vi "AI Block Config Pane.vi"(6 "_SubPanelMessages":refnum<notifier>, 9 "_myEmbeddedToFrameEvent":T7, 10 "_myEmbedded.Exit":refnum<user-event>, 11 "-Property Bundle":cluster{"Name":string, "Value":variant}[](array[cluster])) -> (1 "_Connection Informations":T3, 2 "_Scripter Input":T9)   [LabVIEW 2021]
doc: "Reads values from one or more analog input channels. Use this Express VI to read one or multiple samples for each channel at one time."
uses:
  <vilib>/myRIO/Common/Express VI Framework/xctls/myRIO Channel List/myRIO Channel List.xctl
  <vilib>/myRIO/Common/Express VI Framework/typedefs/Config Pane to Framework Ref.ctl
  <vilib>/myRIO/Common/Express VI Framework/typedefs/Data Validate Ref.ctl
  <vilib>/myRIO/Common/Express VI Framework/typedefs/Scripter Input.ctl
  <vilib>/myRIO/Common/Express VI Framework/typedefs/WireThrough Terminal Names.ctl
  <vilib>/myRIO/Common/Express VI Framework/typedefs/Instrument Driver Method Descriptor Array.ctl
  <vilib>/myRIO/Common/Express VI Framework/typedefs/Instrument Driver Method Descriptor.ctl
  <vilib>/myRIO/Common/Express VI Framework/typedefs/Sub Panel Messages.ctl
  <vilib>/myRIO/Common/Express VI Framework/typedefs/Connection Informations.ctl
  <vilib>/myRIO/Common/Instrument Driver Framework/Utilities/typedefs/Channel Types.ctl
  <vilib>/myRIO/Common/Express VI Framework/vis/Express VI Framework Strings Global.vi
panel:
  in  "Range Indexes":i32[](array[numeric])
  in  "Sample Rate Unit":string="kHz"
  out "_learnMoreLatency":string="Gaps exist between sequential n samples acquisitions. Learn more"
  out "_learnMoreFrequency":string="Detailed information about valid sample rates for this Express VI. Learn more"
  in  "_Validate":bool
  in  "Sample Rate:":dbl=1.0 caption="Sample rate:"
  in  "Samples to Read:":u32=1000 caption="Samples:" min=1 max=10000
  in  "Name:":string="Analog input (n samples)" caption="Node name:"
  in  "Selected Channel List":T1[](xcontrol)=[{"Channel Name"=0, "Channel Alias"="", "Remove Channel"=FALSE, "Index"=0}]
  in  "_Default Alias String":string
  in  "_VI Default Name (Edit and make value default)":string="Analog input (n samples)"
  in  "_WireThrough Info (Edit and make value default)":T4={"WireThrough Top In"="AI (N Samples) Ref In", "WireThrough Bottom In"="error in (no error)", "WireThrough Top Out"="AI (N Samples) Ref Out", "WireThrough Bottom Out"="error out"}
  in  "_Template Array (Edit and make value default)":T5=[{"Function Name"="Smart Open", "VI Path"=path "<vilib>/myRIO/Instrument Drivers/Onboard IO/AI Block/vis", "Script"=TRUE, "Inputs"=[{"name"="Channel Names", "value"=variant, "Config Pane Only"=TRUE, "Build Array"=FALSE, "Bundle Cluster"=FALSE, "Show Term"=FALSE, "alias"=[], "Required Input"=FALSE}], "Outputs"=[], "VI Class"=enum."Open", "Controls Refs[]"=[], "Inline"=FALSE}, {"Function Name"="Open", "VI Path"=path "<vilib>/myRIO/Instrument Drivers/Onboard IO/AI Block/vis", "Script"=FALSE, "Inputs"=[{"name"="Channel Names", "value"=variant, "Config Pane Only"=TRUE, "Build Array"=FALSE, "Bundle Cluster"=FALSE, "Show Term"=FALSE, "alias"=[], "Required Input"=FALSE}], "Outputs"=[], "VI Class"=enum."Open", "Controls Refs[]"=[], "Inline"=FALSE}, {"Function Name"="Read", "VI Path"=path "<vilib>/myRIO/Instrument Drivers/Onboard IO/AI Block/vis", "Script"=TRUE, "Inputs"=[{"name"="Number of Samples", "value"=variant, "Config Pane Only"=TRUE, "Build Array"=FALSE, "Bundle Cluster"=FALSE, "Show Term"=FALSE, "alias"=[], "Required Input"=FALSE}, {"name"="Sample Rate [Hz]", "value"=variant, "Config Pane Only"=TRUE, "Build Array"=FALSE, "Bundle Cluster"=FALSE, "Show Term"=FALSE, "alias"=[], "Required Input"=FALSE}], "Outputs"=[{"name"="Values", "value"=variant, "Show Term"=TRUE, "Index Array"=TRUE, "Unbundle Cluster"=FALSE, "alias"=[]}], "VI Class"=enum."Data", "Controls Refs[]"=[], "Inline"=FALSE}, {"Function Name"="Close", "VI Path"=path "<vilib>/myRIO/Instrument Drivers/Onboard IO/AI Block/vis", "Script"=FALSE, "Inputs"=[], "Outputs"=[], "VI Class"=enum."Close", "Controls Refs[]"=[], "Inline"=FALSE}]
  in  "_Test Close":bool
  # "User Visible Area"
  # "NOTE: Tab Order has been set\nfor this Front Panel.\n1. Name: (string control)\n2. Add Channel (button)\n3. Selected Channel List (array)\n\nAll other controls are excluded \nfrom Tabbing order\n\nTo exlude a control from context\nhelp prefix its label text with a '-'"
  # "kHz"
  # "Gap:"
  # "Acquired signal"
  # "Missed signal"
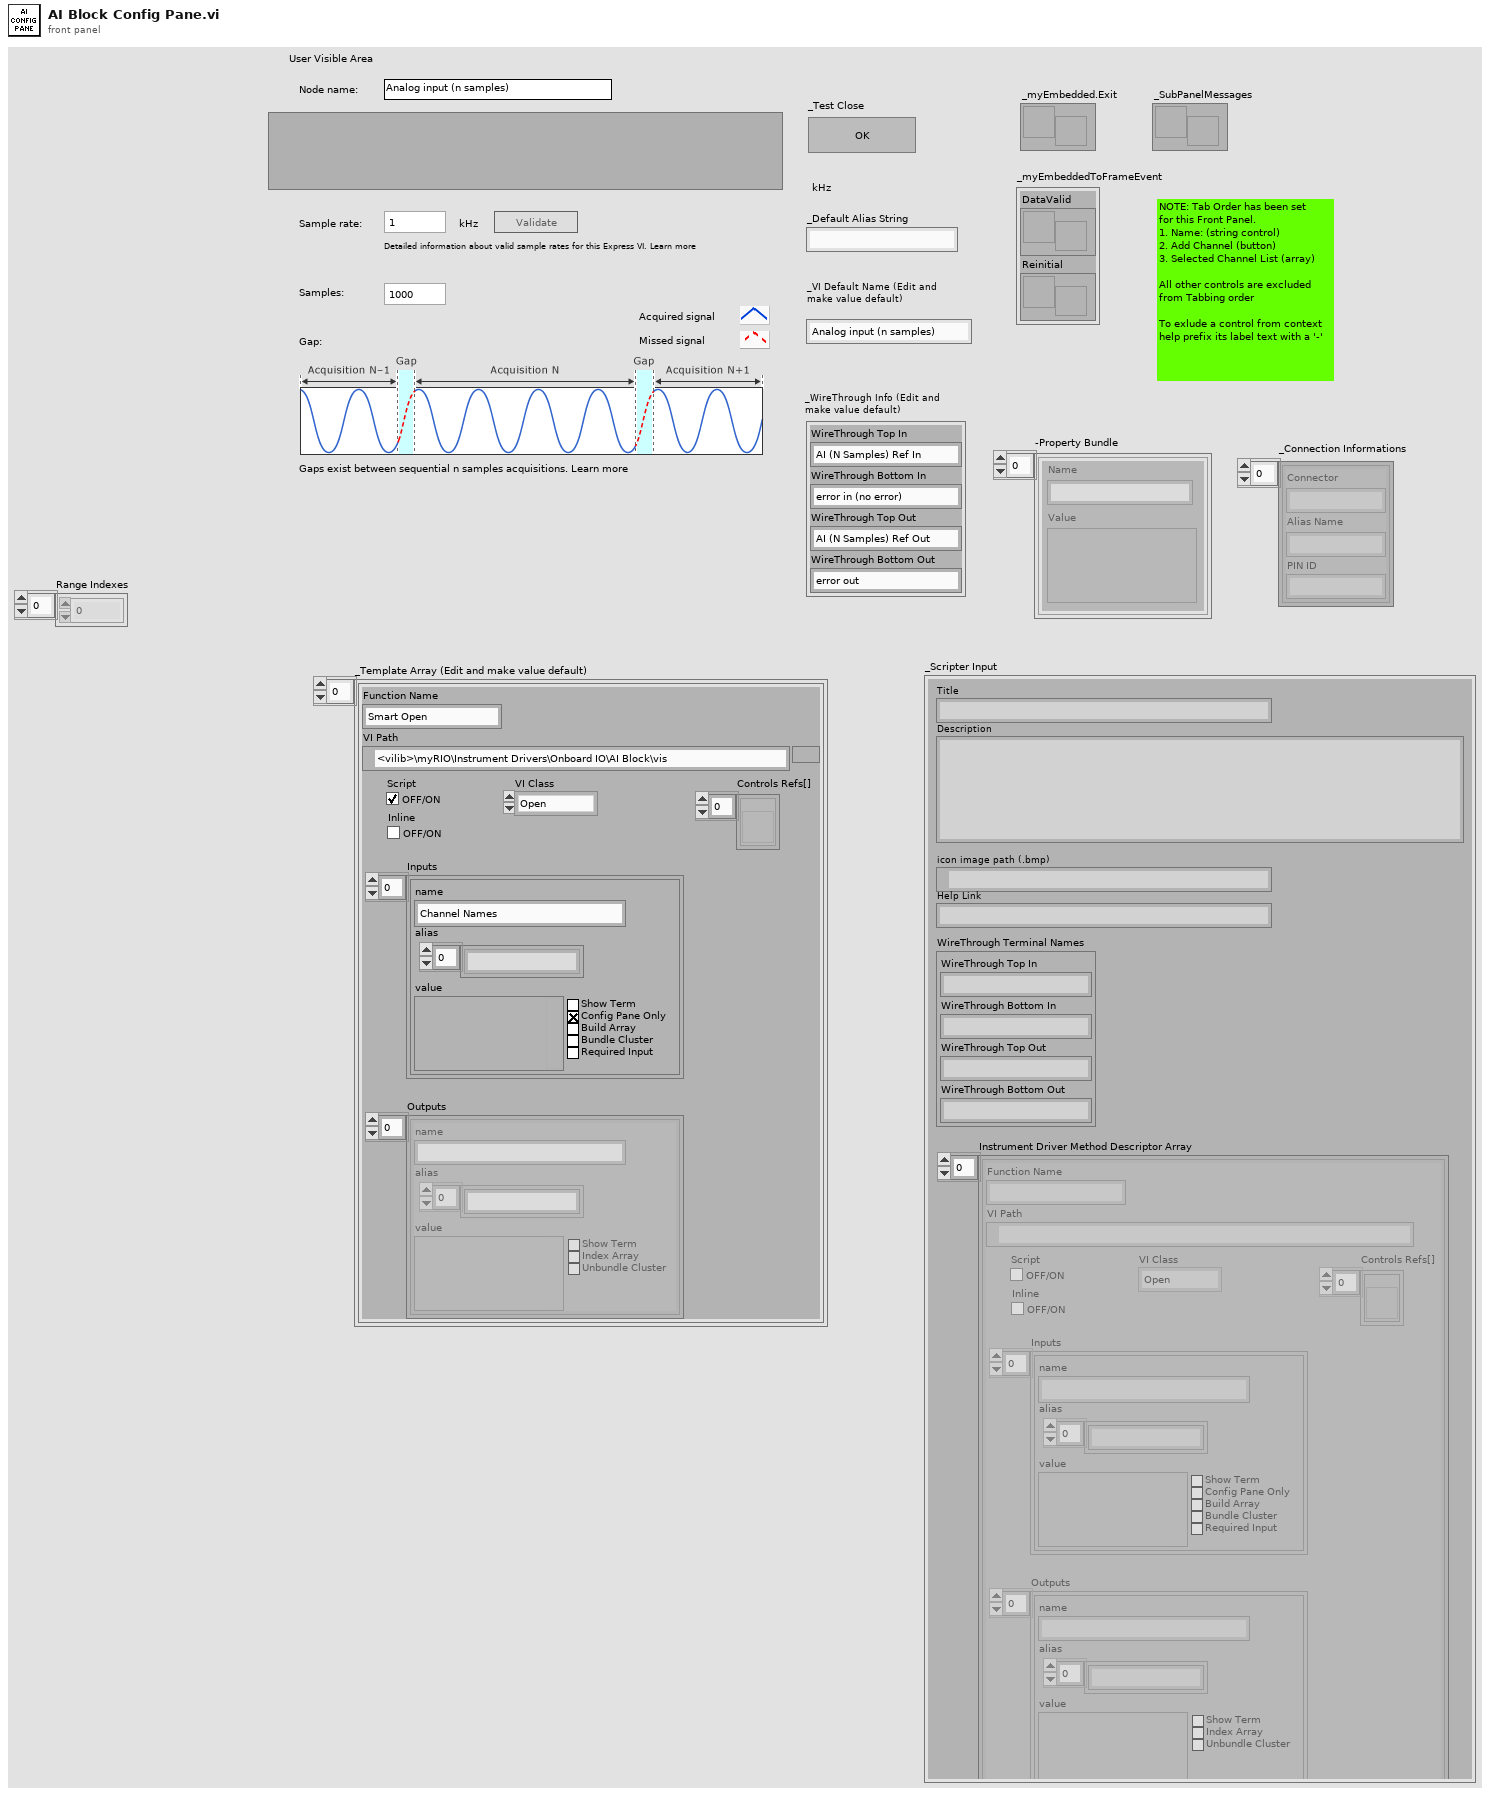
[diagram p1: front panel]
types:
  T1 = typedef "myRIO Channel List.xctl/Channel Data.ctl" = cluster{"Channel Name":u16, "Channel Alias":string, "Remove Channel":T2, "Index":i32}
  T2 = typedef "myRIO Channel List.xctl/Remove Channel.ctl" = bool
  T3 = typedef "Connection Informations.ctl" = cluster{"Connector":string, "Alias Name":string, "PIN ID":string}[]
  T4 = typedef "WireThrough Terminal Names.ctl" = cluster{"WireThrough Top In":string, "WireThrough Bottom In":string, "WireThrough Top Out":string, "WireThrough Bottom Out":string}
  T5 = typedef "Instrument Driver Method Descriptor Array.ctl" = T6[]
  T6 = typedef "Instrument Driver Method Descriptor.ctl" = cluster{"Function Name":string, "VI Path":path, "Script":bool, "Inputs":cluster{"name":string, "value":variant, "Config Pane Only":bool, "Build Array":bool, "Bundle Cluster":bool, "Show Term":bool, "alias":string[], "Required Input":bool}[], "Outputs":cluster{"name":string, "value":variant, "Show Term":bool, "Index Array":bool, "Unbundle Cluster":bool, "alias":string[]}[], "VI Class":enum16{"Open", "Configure", "Data", "Manage", "Close"}, "Controls Refs[]":refnum<vi>[], "Inline":bool}
  T7 = typedef "Config Pane to Framework Ref.ctl" = cluster{"DataValid":T8, "Reinitial":refnum<user-event>}
  T8 = typedef "Data Validate Ref.ctl" = refnum<user-event>
  T9 = typedef "Scripter Input.ctl" = cluster{"Title":string, "Description":string, "icon image path (.bmp)":path, "Help Link":string, "WireThrough Terminal Names":T4, "Instrument Driver Method Descriptor Array":T5}
  T10 = typedef "Channel Types.ctl" = enum32{"Unknown", "AI", "AO", "DIO - DI", "DIO", "DIO - DO", "I2C", "PWM", "Encoder", "SPI", "UART", "Accelerometer", "DIO - LED", "DIO - Button", "AI (N Samples)", "AudioIn (N Samples)", "AO (N Samples)", "AudioOut (N Samples)", "DI (N Samples)", "DO (N Samples)", "AI IRQ", "DI IRQ", "Timer IRQ", "RSL", "Relay", "CAN", "AI (Continuous)", "AO (Continuous)"}
  T11 = typedef "Channel Info.ctl" = cluster{"Channel Name":string, "Alias":string, "Used?":bool, "Not Support?":bool, "Property Bundle":cluster{"Name":string, "Value":variant}[]}
  T12 = typedef "Sub Panel Messages.ctl" = enum16{"Initialized"}
  T13 = enum8{"Enabled", "Disabled", "Disabled and Grayed Out"}
  T14 = cluster{"name":string, "value":variant, "Config Pane Only":bool, "Build Array":bool, "Bundle Cluster":bool, "Show Term":bool, "alias":string[], "Required Input":bool}
  T15 = cluster{"Connector":string, "Alias Name":string, "PIN ID":string}[]
  T16 = cluster{"name":string, "value":variant, "Config Pane Only":bool, "Build Array":bool, "Bundle Cluster":bool, "Show Term":bool, "alias":string[], "Required Input":bool}[]
  T17 = cluster{"name":string, "value":variant, "Show Term":bool, "Index Array":bool, "Unbundle Cluster":bool, "alias":string[]}[]
  T18 = cluster{"name":string, "value":variant, "Show Term":bool, "Index Array":bool, "Unbundle Cluster":bool, "alias":string[]}
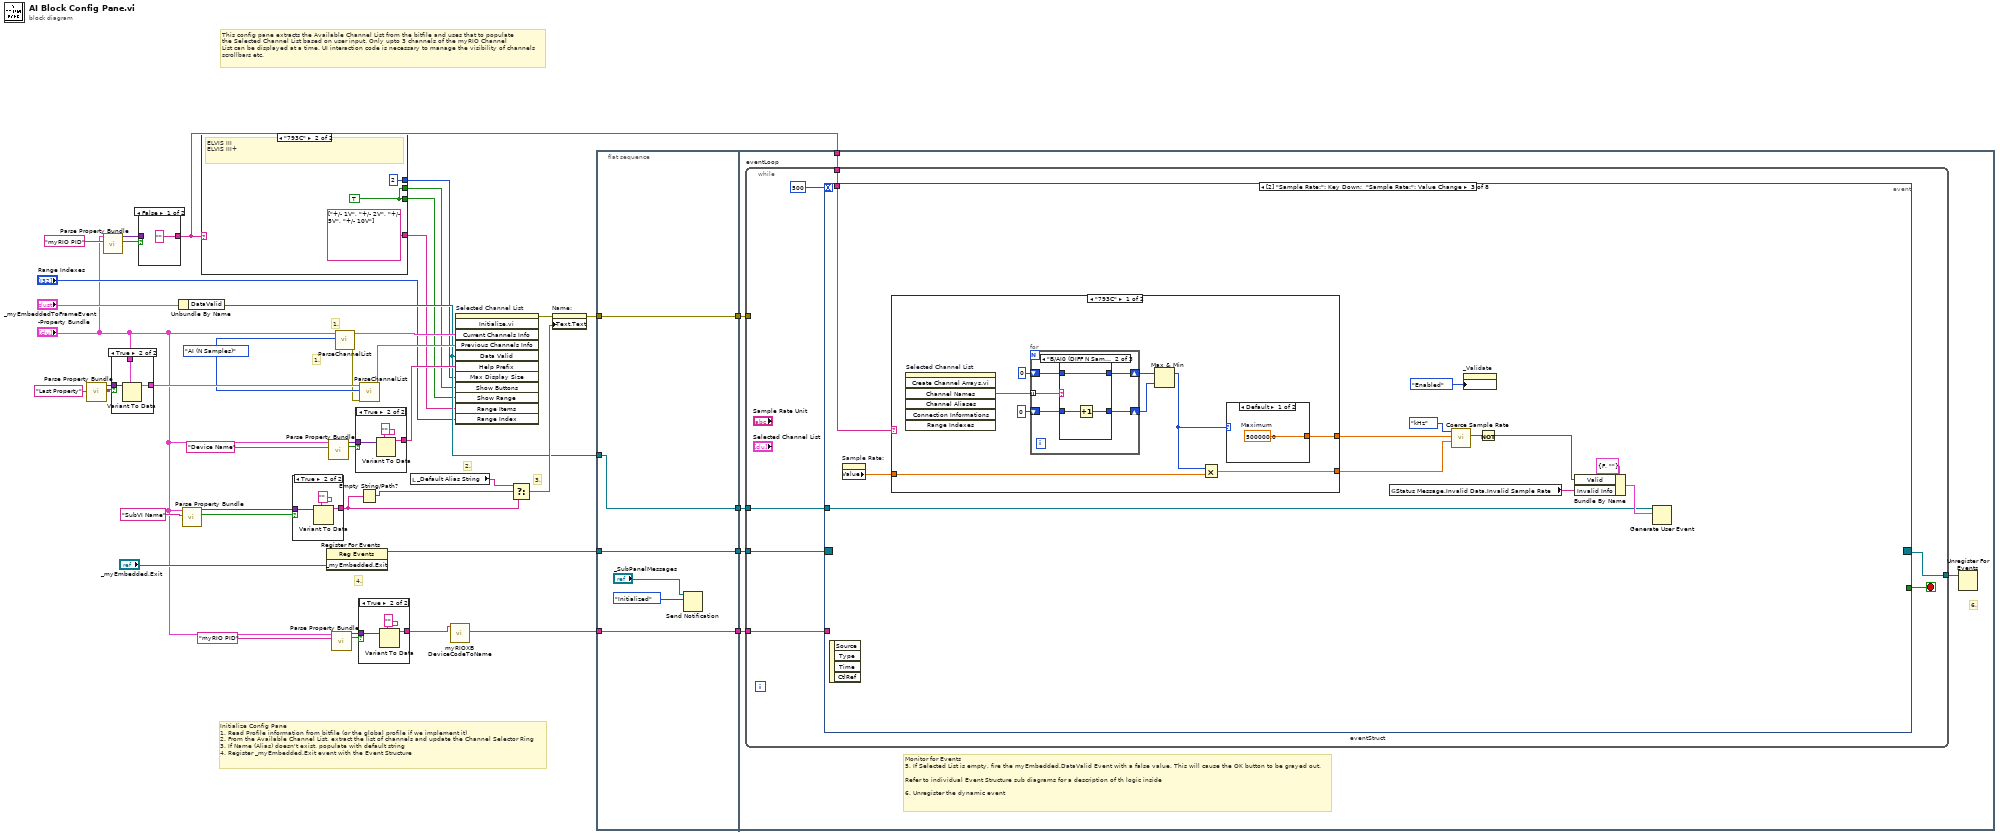
[diagram p0: block diagram]
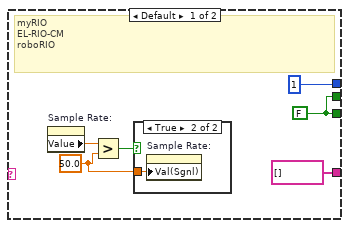
[diagram p2: hidden frame]
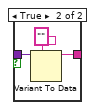
[diagram p4: hidden frame]
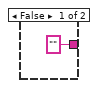
[diagram p5: hidden frame]
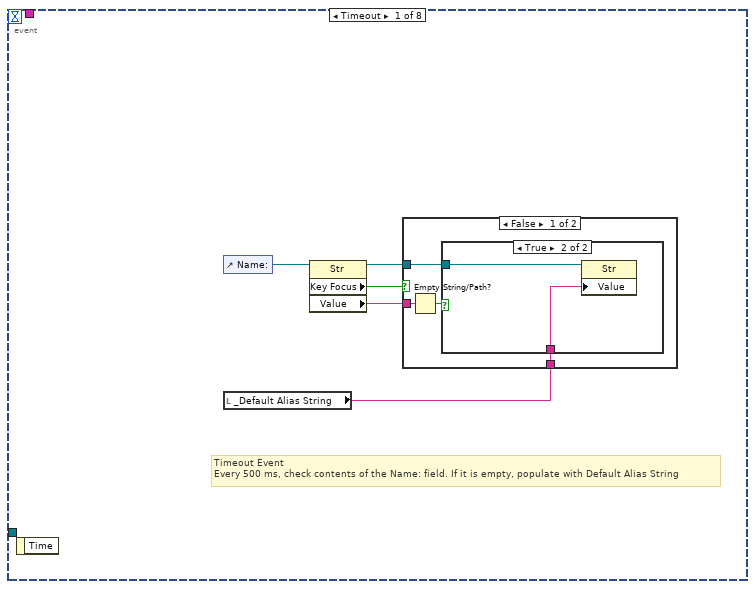
[diagram p6: hidden frame]
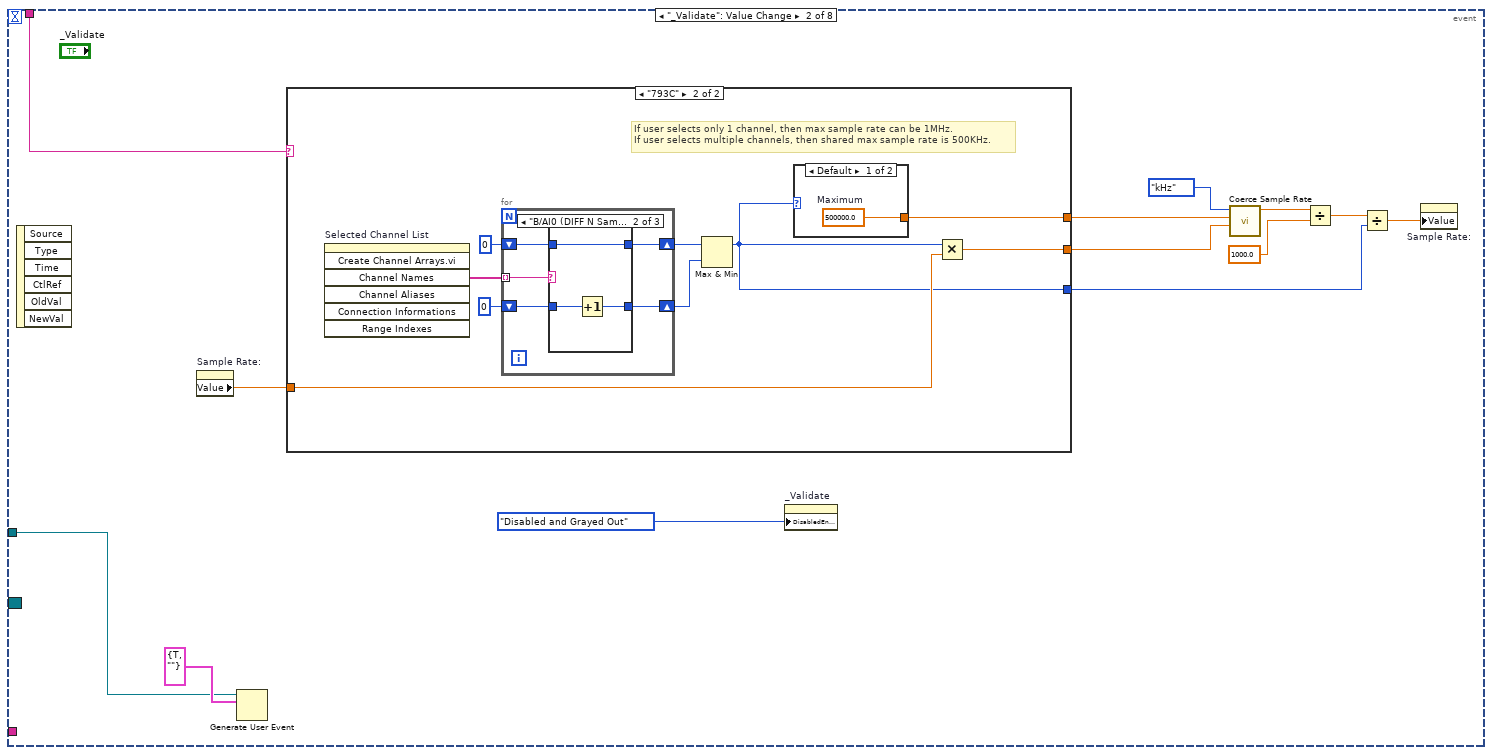
[diagram p9: hidden frame]
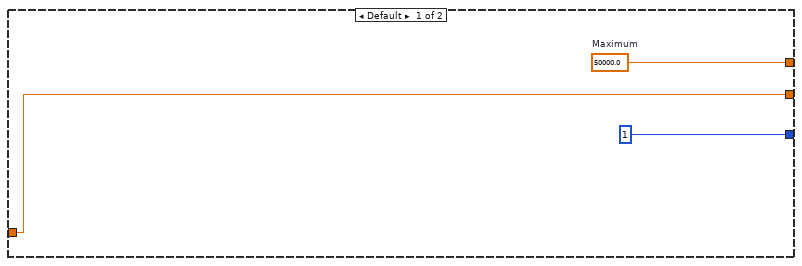
[diagram p10: hidden frame]
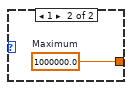
[diagram p11: hidden frame]
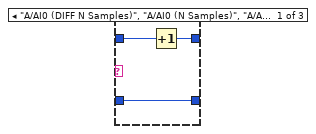
[diagram p12: hidden frame]
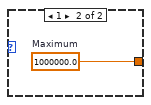
[diagram p14: hidden frame]
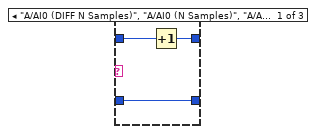
[diagram p15: hidden frame]
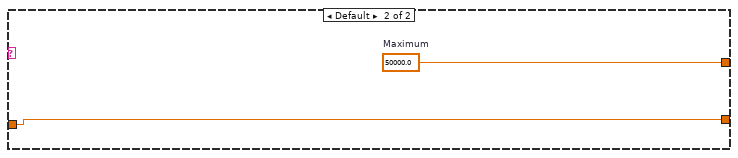
[diagram p17: hidden frame]
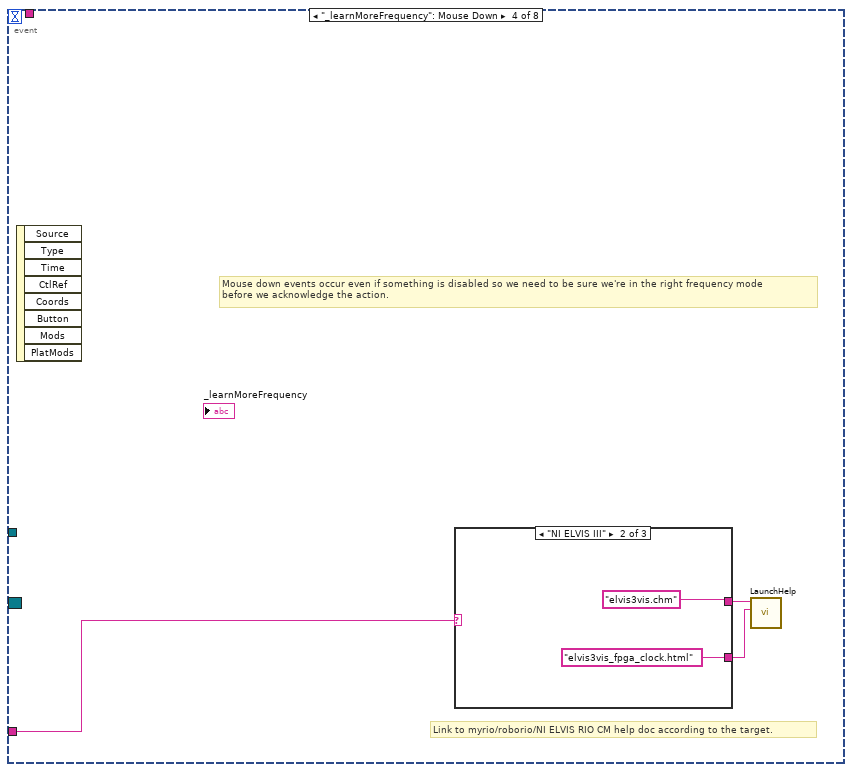
[diagram p18: hidden frame]
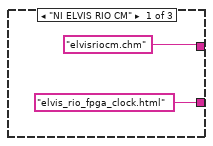
[diagram p19: hidden frame]
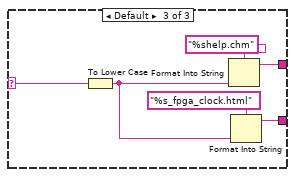
[diagram p20: hidden frame]
diagram:
  w28 = Channel_Types."AI (N Samples)" ("Channel to Read")
  # "1."
  # "2."
  # "1."
  # "This config pane extracts the Available Channel List from the bitfile and uses that to populate\nthe Selected Channel List based on user input. Only upto 3 channels of the myRIO Channel \nList can be displayed at a time. UI interaction code is necessary to manage the visibility of channels\nscrollbars etc."
  # "4."
  # "3."
  # "Initialize Config Pane\n1. Read Profile information from bitfile (or the global profile if we implement it)\n2. From the Available Channel List, extract the list of channels and update the Channel Selector Ring\n3. If Name (Alias) doesn't exist, populate with default string\n4. Register _myEmbedded.Exit event with the Event Structure"
  n1 = call <vilib>:"Parse Property Bundle.vi"("Name"="Last Property") -> ("Found?"=w30:bool, "Value"=w31:variant)  [unwired: 9 in]
  n2 = call <vilib>:"Parse Property Bundle.vi"("Name"="myRIO PID", "Property Bundle"="-Property Bundle") -> ("Found?"=w8:bool, "Value"=w9:variant)  [unwired: 8 in]
  n3 = case shown="True" w30 {
    tunnel: w31 -> [_ w47]
    tunnel: [_ w46] -> w29
    tunnel: "-Property Bundle" -> [_ w45]
    frame False {
    }
    frame True {
      n4 = Variant To Data(type=w45, Variant=w47) -> (data=w46:cluster{"Name":string, "Value":variant}[])  [unwired: 1 in, 1 out]
    }
  }
  n5 = case shown="False" w8 {
    tunnel: w9 -> [_ w51]
    tunnel: ["" ("Name") w50] -> w4
    frame False {
    }
    frame True {
      n6 = Variant To Data(type="" ("Name"), Variant=w51) -> (data=w50:string)  [unwired: 1 in, 1 out]
    }
  }
  n7 = Unbundle By Name("_myEmbeddedToFrameEvent") -> ("DataValid"=w18:T8)
  n8 = call <vilib>:"Parse Property Bundle.vi"("Name"="SubVI Name", "Property Bundle"="-Property Bundle") -> ("Found?"=w38:bool, "Value"=w39:variant)  [unwired: 8 in]
  n9 = case shown="\"793C\"" w4 {
    tunnel: [w56 w60] -> w6
    tunnel: [string[] [] ("Range Items") string[] ["+/- 1V", "+/- 2V", "+/- 5V", "+/- 10V"] ("Range Items")] -> w5
    tunnel: [w56 w60] -> w2
    tunnel: [1 ("Max Display Size") 2 ("Max Display Size")] -> w1
    frame Default {
      w52 = 50.0 ("y")
      w56 = FALSE
      # "myRIO\nEL-RIO-CM\nroboRIO"
      n10 = property on="Sample Rate:" class="DigNum (strict)"() -> ("Value"=w54:dbl)  [unwired: 2 in, 2 out]
      n11 = Greater?(x=w54, y=w52) -> (0:w53:bool)
      n12 = case shown="True" w53 {
        tunnel: w52 -> [_ w58]
        frame False {
        }
        frame True {
          n13 = property on="Sample Rate:" class="DigNum (strict)"("Val(Sgnl)"=w58) -> ()  [unwired: 2 in, 2 out]
        }
      }
    }
    frame "793C" {
      w60 = TRUE
      # "ELVIS III\nELVIS III+"
    }
  }
  n14 = case shown="True" w38 {
    tunnel: w39 -> [_ w65]
    tunnel: ["" ("Name") w63] -> w37
    frame False {
    }
    frame True {
      n15 = Variant To Data(type="" ("Name"), Variant=w65) -> (data=w63:string)  [unwired: 1 in, 1 out]
    }
  }
  n16 = register-events("_myEmbedded.Exit") -> (reference out=w36:refnum<event-registration>)  [unwired: 2 in, 1 out]
  n17 = call <vilib>:"Parse Property Bundle.vi"("Name"="Device Name", "Property Bundle"="-Property Bundle") -> ("Found?"=w24:bool, "Value"=w23:variant)  [unwired: 8 in]
  n18 = call <vilib>:"Parse Property Bundle.vi"("Name"="myRIO PID", "Property Bundle"="-Property Bundle") -> ("Found?"=w14:bool, "Value"=w15:variant)  [unwired: 8 in]
  n19 = call <vilib>:"ParseChannelList.vi"("Channel to Read"=w28, "_Property Bundle"="-Property Bundle") -> ("error out"=w27:errorcluster, "Channel List Out"=w35:T11[])  [unwired: 7 in, 1 out]
  n20 = case shown="True" w24 {
    tunnel: w23 -> [_ w69]
    tunnel: ["" ("Name") w67] -> w21
    frame False {
    }
    frame True {
      n21 = Variant To Data(type="" ("Name"), Variant=w69) -> (data=w67:string)  [unwired: 1 in, 1 out]
    }
  }
  n22 = case shown="True" w14 {
    tunnel: w15 -> [_ w73]
    tunnel: ["" ("Name") w71] -> w12
    frame False {
    }
    frame True {
      n23 = Variant To Data(type="" ("Name"), Variant=w73) -> (data=w71:string)  [unwired: 1 in, 1 out]
    }
  }
  n24 = Empty String/Path?(string/path=w37) -> (empty?=w43:bool)
  n25 = call <vilib>:"ParseChannelList.vi"("error in (no error)"=w27, "Channel to Read"=w28, "_Property Bundle"=w29) -> ("Channel List Out"=w26:T11[])  [unwired: 6 in, 2 out]
  n26 = local read "_Default Alias String"() -> (w33:string)
  n27 = call <vilib>:"myRIOXB DeviceCodeToName.vi"("Device Code"=w12) -> ("Name"=w11:string)  [unwired: 10 in]
  n28 = invoke on="Selected Channel List" class="myRIO Channel List (strict)" method="Initialize.vi"("Current Channels Info"=w35, "Previous Channels Info"=w26, "Data Valid"=w18, "Help Prefix"=w21, "Max Display Size"=w1, "Show Buttons"=w2, "Show Range"=w6, "Range Items"=w5, "Range Index"="Range Indexes") -> (error out=w34:errorcluster)  [unwired: 3 in, 11 out]
  n29 = Select(t=w33, s=w43, f=w37) -> (s? t:f=w42:string)
  n30 = property on="Name:" class="Str"(error in=w34, "Text.Text"=w42) -> (error out=w41:errorcluster)  [unwired: 1 in, 1 out]
  n31 = flat-sequence {
    tunnel: w36 -> [w78]
    tunnel: w41 -> [w79]
    tunnel: [w79] -> w20
    tunnel: [w78] -> w19
    tunnel: w18 -> [w75]
    tunnel: [w75] -> w17
    tunnel: w11 -> [w74]
    tunnel: [w74] -> w13
    tunnel: w20 -> [w84]
    tunnel: w19 -> [w83]
    tunnel: w17 -> [w82]
    tunnel: w13 -> [w81]
    tunnel: w4 -> [w80]
    frame #0 {
      n32 = Send Notification(notification=Sub_Panel_Messages."Initialized", notifier="_SubPanelMessages") -> ()  [unwired: 1 in, 2 out]
    }
    frame #1 {
      # "Monitor for Events\n5. If Selected List is empty, fire the myEmbedded.DataValid Event with a false value. This will cause the OK button to be grayed out.\n\nRefer to individual Event Structure sub diagrams for a description of th logic inside\n\n6. Unregister the dynamic event"
      # "6."
      n33 = while "eventLoop" {
        tunnel: w83 -> [w91]
        tunnel: [w90] -> w85
        tunnel: w84 -> [_]
        tunnel: w82 -> [w88]
        tunnel: w81 -> [w87]
        tunnel: w80 -> [w86]
        stop <- w92 stop-if-true
        n34 = event "eventStruct" shown="[2] \"Sample Rate:\": Key Down;  \"Sample Rate:\": Value Change" {
          selector: w91 -> [_ _ _ _ _ _ _ _]
          dyn-events: [_ _ _ _ _ _ _ _] -> w90
          timeout: 500 -> [_ _ _ _ _ _ _ _]
          tunnel: [_ _ _ _ _ TRUE ("_Test Close") _ _] -> w92
          tunnel: w88 -> [_ w114 w151 _ _ _ _ _]
          tunnel: w87 -> [_ _ _ w182 _ _ _ _]
          tunnel: w86 -> [_ w113 w147 _ _ w203 _ _]
          event Timeout {
            # "Timeout Event\nEvery 500 ms, check contents of the Name: field. If it is empty, populate with Default Alias String"
            n35 = event-data() -> ()  [unwired: 1 in, 1 out]
            n36 = control-ref of="Name:"() -> (w95:refnum<vi>)
            n37 = local read "_Default Alias String"() -> (w93:string)
            n38 = property on="Property Node" class="Str"(reference=w95) -> (reference out=w94:refnum<vi>, "Key Focus"=w96:bool, "Value"=w97:string)  [unwired: 1 in, 1 out]
            n39 = case shown="False" w96 {
              tunnel: w97 -> [w101 _]
              tunnel: w94 -> [w99 _]
              tunnel: w93 -> [w98 _]
              frame False {
                n40 = Empty String/Path?(string/path=w101) -> (empty?=w100:bool)
                n41 = case shown="True" w100 {
                  tunnel: w99 -> [_ w103]
                  tunnel: w98 -> [_ w102]
                  frame False {
                  }
                  frame True {
                    n42 = property on="Property Node" class="Str"(reference=w103, "Value"=w102) -> ()  [unwired: 1 in, 2 out]
                  }
                }
              }
              frame True {
              }
            }
          }
          event "_Validate": Value Change {
            n43 = event-data() -> ()  [unwired: 1 in, 6 out]
            n44 = property on="Sample Rate:" class="DigNum (strict)"() -> ("Value"=w112:dbl)  [unwired: 2 in, 2 out]
            n45 = Generate User Event(user event=w114, event data cluster=cluster{"Valid":bool, "Invalid Info":string} {"Valid"=TRUE, "Invalid Info"=""} ("event data")) -> ()  [unwired: 2 in, 2 out]
            n46 = case shown="\"793C\"" w113 {
              tunnel: w112 -> [w118 w123]
              tunnel: [w118 w122] -> w109
              tunnel: [w119 w121] -> w106
              tunnel: [1 w120] -> w104
              frame Default {
                w119 = 50000.0  # Maximum
              }
              frame "793C" {
                # "If user selects only 1 channel, then max sample rate can be 1MHz.\nIf user selects multiple channels, then shared max sample rate is 500KHz."
                n47 = invoke on="Selected Channel List" class="myRIO Channel List (strict)" method="Create Channel Arrays.vi"() -> ("Channel Names"=w128:string[])  [unwired: 7 in, 6 out]
                n48 = for {
                  tunnel: w128 -> [w135] mode=indexing
                  shift-right: [w133] -> w125
                  shift-left: 0 -> [w134]
                  shift-right: [w131] -> w124
                  shift-left: 0 -> [w132]
                  n49 = case shown="\"B/AI0 (DIFF N Samples)\", \"B/AI0 (N Samples)\", \"B/AI1 (DIFF N Samples)\", \"B/AI1 (N Samples)\", \"B/AI2 (DIFF N Samples)\", \"B/AI2 (N Samples)\", \"B/AI3 (DIFF N Samples)\", \"B/AI3 (N Samples)\", \"B/AI4 (N Samples)\", \"B/AI5 (N Samples)\", \"B/AI6 (N Samples)\", \"B/AI7 (N Samples)\"" w135 {
                    tunnel: w134 -> [w138 w141 w143]
                    tunnel: [w137 w141 w143] -> w133
                    tunnel: w132 -> [w136 w140 w142]
                    tunnel: [w136 w139 w142] -> w131
                    frame "A/AI0 (DIFF N Samples)", "A/AI0 (N Samples)", "A/AI1 (DIFF N Samples)", "A/AI1 (N Samples)", "A/AI2 (DIFF N Samples)", "A/AI2 (N Samples)", "A/AI3 (DIFF N Samples)", "A/AI3 (N Samples)", "A/AI4 (N Samples)", "A/AI5 (N Samples)", "A/AI6 (N Samples)", "A/AI7 (N Samples)" {
                      n50 = Increment(x=w138) -> (x+1=w137:i32)
                    }
                    frame "B/AI0 (DIFF N Samples)", "B/AI0 (N Samples)", "B/AI1 (DIFF N Samples)", "B/AI1 (N Samples)", "B/AI2 (DIFF N Samples)", "B/AI2 (N Samples)", "B/AI3 (DIFF N Samples)", "B/AI3 (N Samples)", "B/AI4 (N Samples)", "B/AI5 (N Samples)", "B/AI6 (N Samples)", "B/AI7 (N Samples)" {
                      n51 = Increment(x=w140) -> (x+1=w139:i32)
                    }
                    frame Default {
                    }
                  }
                }
                n52 = Max & Min(x=w125, y=w124) -> (max(x,y)=w120:i32)  [unwired: 1 out]
                n53 = case shown="Default" w120 {
                  tunnel: [w129 w130] -> w121
                  frame Default {
                    w129 = 500000.0  # Maximum
                  }
                  frame 1 {
                    w130 = 1000000.0  # Maximum
                  }
                }
                n54 = Multiply(x=w120, y=w123) -> (x*y=w122:dbl)
              }
            }
            n55 = property on="_Validate" class="Bool"("DisabledEnum"=T13."Disabled and Grayed Out" ("Disabled")) -> ()  [unwired: 2 in, 2 out]
            n56 = call <vilib>:"Coerce Sample Rate.vi"("Sample Rate:"=w109, "Maximum"=w106, "Sample Rate Unit"=enum16{"Hz", "kHz", "MHz"}."kHz") -> ("Actual Sample Rate (s)"=w111:dbl)  [unwired: 7 in, 1 out]
            n57 = Divide(x=w111, y=1000.0) -> (x/y=w107:dbl)
            n58 = Divide(x=w107, y=w104) -> (x/y=w105:dbl)
            n59 = property on="Sample Rate:" class="DigNum (strict)"("Value"=w105) -> ()  [unwired: 2 in, 2 out]
          }
          event "Sample Rate:": Key Down; "Sample Rate:": Value Change {
            n60 = event-data() -> ()  [unwired: 1 in, 4 out]
            n61 = property on="Sample Rate:" class="DigNum (strict)"() -> ("Value"=w145:dbl)  [unwired: 2 in, 2 out]
            n62 = case shown="\"793C\"" w147 {
              tunnel: [w157 w181] -> w146
              tunnel: w145 -> [w159 w180]
              tunnel: [w158 w180] -> w144
              frame "793C" {
                n63 = invoke on="Selected Channel List" class="myRIO Channel List (strict)" method="Create Channel Arrays.vi"() -> ("Channel Names"=w162:string[])  [unwired: 7 in, 6 out]
                n64 = for {
                  tunnel: w162 -> [w171] mode=indexing
                  shift-right: [w169] -> w163
                  shift-left: 0 -> [w170]
                  shift-right: [w167] -> w164
                  shift-left: 0 -> [w168]
                  n65 = case shown="\"B/AI0 (DIFF N Samples)\", \"B/AI0 (N Samples)\", \"B/AI1 (DIFF N Samples)\", \"B/AI1 (N Samples)\", \"B/AI2 (DIFF N Samples)\", \"B/AI2 (N Samples)\", \"B/AI3 (DIFF N Samples)\", \"B/AI3 (N Samples)\", \"B/AI4 (N Samples)\", \"B/AI5 (N Samples)\", \"B/AI6 (N Samples)\", \"B/AI7 (N Samples)\"" w171 {
                    tunnel: w170 -> [w174 w177 w179]
                    tunnel: [w173 w177 w179] -> w169
                    tunnel: w168 -> [w172 w176 w178]
                    tunnel: [w172 w175 w178] -> w167
                    frame "A/AI0 (DIFF N Samples)", "A/AI0 (N Samples)", "A/AI1 (DIFF N Samples)", "A/AI1 (N Samples)", "A/AI2 (DIFF N Samples)", "A/AI2 (N Samples)", "A/AI3 (DIFF N Samples)", "A/AI3 (N Samples)", "A/AI4 (N Samples)", "A/AI5 (N Samples)", "A/AI6 (N Samples)", "A/AI7 (N Samples)" {
                      n66 = Increment(x=w174) -> (x+1=w173:i32)
                    }
                    frame "B/AI0 (DIFF N Samples)", "B/AI0 (N Samples)", "B/AI1 (DIFF N Samples)", "B/AI1 (N Samples)", "B/AI2 (DIFF N Samples)", "B/AI2 (N Samples)", "B/AI3 (DIFF N Samples)", "B/AI3 (N Samples)", "B/AI4 (N Samples)", "B/AI5 (N Samples)", "B/AI6 (N Samples)", "B/AI7 (N Samples)" {
                      n67 = Increment(x=w176) -> (x+1=w175:i32)
                    }
                    frame Default {
                    }
                  }
                }
                n68 = Max & Min(x=w163, y=w164) -> (max(x,y)=w156:i32)  [unwired: 1 out]
                n69 = Multiply(x=w156, y=w159) -> (x*y=w158:dbl)
                n70 = case shown="Default" w156 {
                  tunnel: [w165 w166] -> w157
                  frame Default {
                    w165 = 500000.0  # Maximum
                  }
                  frame 1 {
                    w166 = 1000000.0  # Maximum
                  }
                }
              }
              frame Default {
                w181 = 50000.0  # Maximum
              }
            }
            n71 = global read "Express VI Framework Strings Global.vi" "Status Message.Invalid Data.Invalid Sample Rate"() -> (w152:string)
            n72 = call <vilib>:"Coerce Sample Rate.vi"("Sample Rate:"=w144, "Maximum"=w146, "Sample Rate Unit"=enum16{"Hz", "kHz", "MHz"}."kHz") -> ("Coercion needed?"=w149:bool)  [unwired: 7 in, 1 out]
            n73 = property on="_Validate" class="Bool"("DisabledEnum"=T13."Enabled" ("Disabled")) -> ()  [unwired: 2 in, 2 out]
            n74 = Not(x=w149) -> (.not. x?=w148:bool)
            n75 = Bundle By Name(cluster=cluster{"Valid":bool, "Invalid Info":string} {"Valid"=FALSE, "Invalid Info"=""} ("event data"), "Valid"=w148, "Invalid Info"=w152) -> (w153:cluster{"Valid":bool, "Invalid Info":string})
            n76 = Generate User Event(user event=w151, event data cluster=w153) -> ()  [unwired: 2 in, 2 out]
          }
          event "_learnMoreFrequency": Mouse Down {
            # "Link to myrio/roborio/NI ELVIS RIO CM help doc according to the target."
            # "Mouse down events occur even if something is disabled so we need to be sure we're in the right frequency mode\nbefore we acknowledge the action."
            n77 = event-data() -> ()  [unwired: 1 in, 8 out]
            n78 = case shown="\"NI ELVIS III\"" w182 {
              selector: w182 -> [_ _ w189]
              tunnel: ["elvisriocm.chm" ("Help File") "elvis3vis.chm" ("Help File") w191] -> w184
              tunnel: ["elvis_rio_fpga_clock.html" ("Help Topic") "elvis3vis_fpga_clock.html" ("Help Topic") w190] -> w183
              frame "NI ELVIS RIO CM" {
              }
              frame "NI ELVIS III" {
              }
              frame Default {
                n79 = To Lower Case(string=w189) -> (all lower case string=w193:string)
                n80 = Format Into String(format string="%shelp.chm" ("Help File"), w193) -> (resulting string=w191:string)  [unwired: 2 in, 1 out]
                n81 = Format Into String(format string="%s_fpga_clock.html" ("Help Topic"), w193) -> (resulting string=w190:string)  [unwired: 2 in, 1 out]
              }
            }
            n82 = call <vilib>:"LaunchHelp.vi"("Help Topic"=w183, "Help File"=w184) -> ()  [unwired: 10 in]
          }
          event "Name:": Mouse Down {
            # "If Mouse Down event is generated by the Name: Control,\ncheck if value == Default Alias String, if yes, replace with null string"
            n83 = event-data() -> ("CtlRef"=w201:refnum<vi>)  [unwired: 1 in]
            n84 = local read "_Default Alias String"() -> (w195:string)
            n85 = property class="Str"(reference=w201) -> (reference out=w197:refnum<vi>, "Value"=w196:string)  [unwired: 1 in, 1 out]
            n86 = Equal?(x=w196, y=w195) -> (x = y?=w200:bool)
            n87 = Select(t="", s=w200, f=w196) -> (s? t:f=w198:string)
            n88 = property class="Str"(reference=w197, "Value"=w198) -> ()  [unwired: 1 in, 2 out]
          }
          event User Event; "_Test Close": Value Change {
            # "2."
            # "1."
            # "1. Create array of all Channel Aliases and wire it out to the alias array for the appropriate output\n2. Create array of all Channel Names and wire it out to the Channel Names input\n3. Ensure that Template IDM array has correct Instrument Driver information and update appropriate fields\n4. If user has not created custom name (alias) for VI, then use VI Default Name"
            # "4."
            # "3."
            # "Pass node strings to framework for scripting.\n- Title appears under icon on Express VI node.\n- Description appears in context help."
            n89 = event-data() -> ()  [unwired: 1 in, 1 out]
            n90 = case shown="\"793C\"" w203 {
              tunnel: [w228 w229] -> w202
              frame "793C" {
                w228 = 1000000.0  # Maximum
              }
              frame Default {
                w229 = 50000.0  # Maximum
              }
            }
            n91 = invoke on="Selected Channel List" class="myRIO Channel List (strict)" method="Create Channel Arrays.vi"() -> ("Channel Names"=w211:string[], "Channel Aliases"=w210:string[], "Connection Informations"=→"_Connection Informations":T15, "Range Indexes"=w204:i32[])  [unwired: 7 in, 3 out]
            n92 = call <vilib>:"Coerce Sample Rate.vi"("Sample Rate:"="Sample Rate:", "Maximum"=w202, "Sample Rate Unit"=enum16{"Hz", "kHz", "MHz"}."kHz") -> ("Actual Sample Rate (s)"=w207:dbl)  [unwired: 7 in, 1 out]
            n93 = in-place {
              in-place-border: w211 -> [w236]
              in-place-border: w210 -> [w235]
              in-place-border: "Samples to Read:" -> [w233]
              in-place-border: w207 -> [w232]
              in-place-border: w204 -> [w231]
              in-place-border: w203 -> [w230]
              n94 = in-place-array #1("_Template Array (Edit and make value default)", 0, 2) -> (w239:T6, w234:T6)
              n95 = in-place {
                in-place-border: w236 -> [w268]
                in-place-border: w231 -> [w266]
                in-place-border: w230 -> [w265]
                n96 = in-place-cluster #2(w239) -> ("Function Name"=w264:string, "Inputs"=w269:T16)
                n97 = in-place {
                  in-place-border: w268 -> [w314]
                  n98 = in-place-array #3(w269, 0) -> (w317:T14)
                  n99 = To Variant(anything=w314) -> (Variant=w315:variant)
                  n100 = Bundle By Name(cluster=w317, "value"=w315) -> (w316:T14)
                  n101 = in-place-array #3(w316) -> (w263:T16)  [unwired: 1 out]
                }
                n102 = case shown="\"793C\"" w265 {
                  tunnel: w264 -> [w271 _]
                  tunnel: [w271 "Smart Open With Range"] -> w262
                  tunnel: w263 -> [w270 w283]
                  tunnel: w266 -> [_ w282]
                  tunnel: [w270 w272] -> w261
                  frame Default {
                    # "myRIO,EL-RIO-CM,roboRIO"
                  }
                  frame "793C" {
                    w281 = dbl[] []
                    # "ELVIS III, ELVIS III+"
                    n103 = for {
                      tunnel: w282 -> [w289] mode=indexing
                      shift-right: [w287] -> w279
                      shift-left: w281 -> [w288]
                      shift-right: [w285] -> w276
                      shift-left: w281 -> [w286]
                      n104 = case shown="1" w289 {
                        tunnel: w288 -> [w293 w299 w305 w311]
                        tunnel: [w292 w298 w304 w310] -> w287
                        tunnel: w286 -> [w291 w297 w303 w309]
                        tunnel: [w290 w296 w302 w308] -> w285
                        frame 0, Default {
                          n105 = Build Array (concatenate)(w293, -1.0) -> (w292:dbl[])
                          n106 = Build Array (concatenate)(w291, 1.0) -> (w290:dbl[])
                        }
                        frame 1 {
                          n107 = Build Array (concatenate)(w299, -2.0) -> (w298:dbl[])
                          n108 = Build Array (concatenate)(w297, 2.0) -> (w296:dbl[])
                        }
                        frame 2 {
                          n109 = Build Array (concatenate)(w305, -5.0) -> (w304:dbl[])
                          n110 = Build Array (concatenate)(w303, 5.0) -> (w302:dbl[])
                        }
                        frame 3 {
                          n111 = Build Array (concatenate)(w311, -10.0) -> (w310:dbl[])
                          n112 = Build Array (concatenate)(w309, 10.0) -> (w308:dbl[])
                        }
                      }
                    }
                    n113 = To Variant(anything=w279) -> (Variant=w280:variant)
                    n114 = To Variant(anything=w276) -> (Variant=w277:variant)
                    n115 = Bundle By Name(cluster=T14 {"name"="Min Value", "value"=variant, "Config Pane Only"=TRUE, "Build Array"=FALSE, "Bundle Cluster"=FALSE, "Show Term"=FALSE, "alias"=[], "Required Input"=FALSE} ("element"), "value"=w280) -> (w274:T14)
                    n116 = Bundle By Name(cluster=T14 {"name"="Max Value", "value"=variant, "Config Pane Only"=TRUE, "Build Array"=FALSE, "Bundle Cluster"=FALSE, "Show Term"=FALSE, "alias"=[], "Required Input"=FALSE} ("element"), "value"=w277) -> (w273:T14)
                    n117 = Build Array (concatenate)(w283, w274, w273) -> (w272:T16)
                  }
                }
                n118 = in-place-cluster #2("Function Name"=w262, "Inputs"=w261) -> (w238:T6)
              }
              n119 = in-place {
                in-place-border: w235 -> [w248]
                in-place-border: w233 -> [w242]
                in-place-border: w232 -> [w241]
                n120 = in-place-cluster #4(w234) -> ("Outputs"=w249:T17, "Inputs"=w245:T16)
                n121 = in-place {
                  in-place-border: w248 -> [w258]
                  n122 = in-place-array #5(w249, 0) -> (w260:T18)
                  n123 = Bundle By Name(cluster=w260, "alias"=w258) -> (w259:T18)
                  n124 = in-place-array #5(w259) -> (w247:T17)  [unwired: 1 out]
                }
                n125 = in-place {
                  in-place-border: w242 -> [w255]
                  in-place-border: w241 -> [w252]
                  n126 = in-place-array #6(w245, 0, 1) -> (w257:T14, w253:T14)
                  n127 = To Variant(anything=w255) -> (Variant=w254:variant)
                  n128 = To Variant(anything=w252) -> (Variant=w251:variant)
                  n129 = Bundle By Name(cluster=w257, "value"=w254) -> (w256:T14)
                  n130 = Bundle By Name(cluster=w253, "value"=w251) -> (w250:T14)
                  n131 = in-place-array #6(w256, w250) -> (w244:T16)  [unwired: 2 out]
                }
                n132 = in-place-cluster #4("Outputs"=w247, "Inputs"=w244) -> (w237:T6)
              }
              n133 = in-place-array #1(w238, w237) -> (w225:T5)  [unwired: 2 out]
            }
            n134 = Divide(x=w207, y=1000.0) -> (x/y=w205:dbl)
            n135 = local write "Range Indexes"(w204) -> ()
            n136 = property on="Sample Rate:" class="DigNum (strict)"("Value"=w205) -> ()  [unwired: 2 in, 2 out]
            n137 = Equal?(x="_Default Alias String", y="Name:") -> (x = y?=w217:bool)
            n138 = Select(t="_VI Default Name (Edit and make value default)", s=w217, f="Name:") -> (s? t:f=w215:string)
            n139 = Bundle By Name(cluster=T9 {"Title"="", "Description"="", "icon image path (.bmp)"=path "", "Help Link"="", "WireThrough Terminal Names"={"WireThrough Top In"="", "WireThrough Bottom In"="", "WireThrough Top Out"="", "WireThrough Bottom Out"=""}, "Instrument Driver Method Descriptor Array"=[]} ("Scripter Input"), "Instrument Driver Method Descriptor Array"=w225, "WireThrough Terminal Names"="_WireThrough Info (Edit and make value default)", "Title"=w215, "Description"="" ("Title")) -> (→"_Scripter Input":T9)
          }
          event "_learnMoreLatency": Mouse Down {
            n140 = event-data() -> ()  [unwired: 1 in, 6 out]
            n141 = call <vilib>:"LaunchHelp.vi"("Help Topic"="myrioref_exp_ai.html#details", "Help File"="myrioreference.chm") -> ()  [unwired: 10 in]
          }
          event "Selected Channel List": Value Change {
            n142 = event-data() -> ("OldVal"=w324:T1[], "NewVal"=w323:T1[])  [unwired: 1 in, 4 out]
            n143 = Array Size(array=w324) -> (size(s)=w322:i32)
            n144 = Array Size(array=w323) -> (size(s)=w321:i32)
            n145 = Not Equal?(x=w322, y=w321) -> (x != y?=w320:bool)
            n146 = case shown="True" w320 {
              frame False {
              }
              frame True {
                n147 = property on="Sample Rate:" class="DigNum (strict)"() -> ("Value"=w325:dbl)  [unwired: 2 in, 2 out]
                n148 = property on="Sample Rate:" class="DigNum (strict)"("Val(Sgnl)"=w325) -> ()  [unwired: 2 in, 2 out]
              }
            }
          }
        }
      }
      n149 = Unregister For Events(event registration refnum=w85) -> ()  [unwired: 1 in, 1 out]
    }
  }
